vi "simpletest.vi"() -> ()   [LabVIEW 2015]
uses:
  inp.vi
  time_logic.vi
panel:
  out "Array 2":string[](array[string])
  out "Array":dbl[](array[numeric])
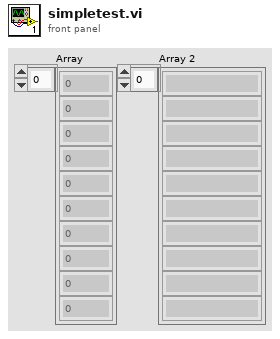
[diagram p1: front panel]
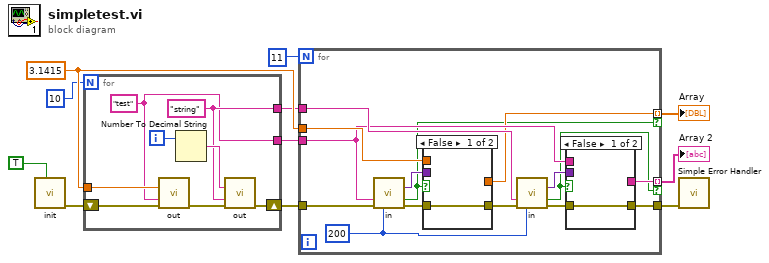
[diagram p0: block diagram]
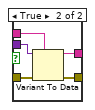
[diagram p2: hidden frame]
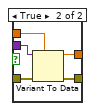
[diagram p3: hidden frame]
diagram:
  w9 = 3.1415
  n1 = call "init.vi"("Cleaneup"=TRUE ("Cleneup")) -> ("error out"=w10:errorcluster)  [unwired: 10 in]
  n2 = for {
    N: 10 -> [_]
    tunnel: w9 -> [w18]
    tunnel: [w14] -> w6
    tunnel: [w13] -> w5
    shift-right: [w16] -> w7
    shift-left: w10 -> [w19]
    i -> [w12]
    w14 = "string" ("Name in")
    w13 = "test" ("Name in")
    n3 = call "out.vi"("IN VARIANT"=w18, "Name in"=w13, "error in (no error)"=w19) -> ("error out"=w17:errorcluster)  [unwired: 11 in, 1 out]
    n4 = Number To Decimal String(number=w12) -> (decimal integer string=w15:string)  [unwired: 1 in]
    n5 = call "out.vi"("IN VARIANT"=w15, "Name in"=w14, "error in (no error)"=w17) -> ("error out"=w16:errorcluster)  [unwired: 11 in, 1 out]
  }
  n6 = for {
    N: 11 -> [_]
    tunnel: w9 -> [w34]
    tunnel: [w33] -> w8 mode=indexing if=w20
    tunnel: w7 -> [w30]
    tunnel: w6 -> [w28]
    tunnel: w5 -> [w26]
    tunnel: [w25] -> w4 mode=indexing if=w21
    tunnel: [w23] -> w1
    w22 = 200 ("timout")
    n7 = call "in.vi"("Name in"=w26, "error in (no error)"=w30, "timout"=w22) -> ("OUT VARIANT"=w32:variant, "Valid data"=w21:bool, "error out"=w31:errorcluster)  [unwired: 10 in]
    n8 = case shown="False" w21 {
      tunnel: w34 -> [_ w46]
      tunnel: w32 -> [_ w45]
      tunnel: w31 -> [w41 w44]
      tunnel: [w41 w43] -> w29
      tunnel: [_ w42] -> w25
      frame False {
      }
      frame True {
        n9 = Variant To Data(error in=w44, type=w46, Variant=w45) -> (data=w42:dbl, error out=w43:errorcluster)
      }
    }
    n10 = call "in.vi"("Name in"=w28, "error in (no error)"=w29, "timout"=w22) -> ("OUT VARIANT"=w27:variant, "Valid data"=w20:bool, "error out"=w24:errorcluster)  [unwired: 10 in]
    n11 = case shown="False" w20 {
      tunnel: [_ w40] -> w33
      tunnel: w27 -> [_ w39]
      tunnel: w26 -> [_ w38]
      tunnel: w24 -> [w35 w37]
      tunnel: [w35 w36] -> w23
      frame False {
      }
      frame True {
        n12 = Variant To Data(error in=w37, type=w38, Variant=w39) -> (data=w40:string, error out=w36:errorcluster)
      }
    }
  }
  "Array 2" <- w8
  "Array" <- w4
  n13 = call <vilib>:"Simple Error Handler.vi"("error in (no error)"=w1) -> ()  [unwired: 4 in, 5 out]
